vi "Get Named Range.vi"(7 "Sheet Name":string, 8 "error in":errorcluster, 10 "Range Identifier":string, 11 "SpreadsheetDoc in":refnum<k24>) -> (0 "error out":errorcluster, 2 "Range":string, 3 "SpreadsheetDoc out":refnum<k24>, 5 "Sheet Name":string)   [LabVIEW 2019, in "Open Xml.lvlib"]
uses:
  Open Xml.lvlib
  D:/git/Open-Xml-LabVIEW/Source/DocumentFormat.OpenXml.dll
  DocumentFormat.OpenXml.dll
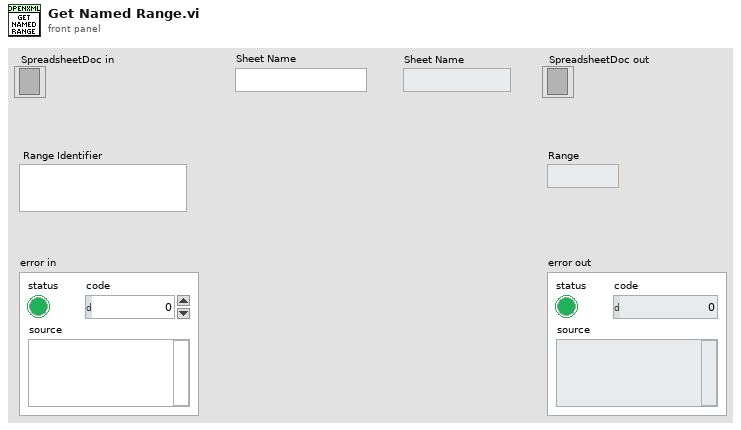
[diagram p1: front panel]
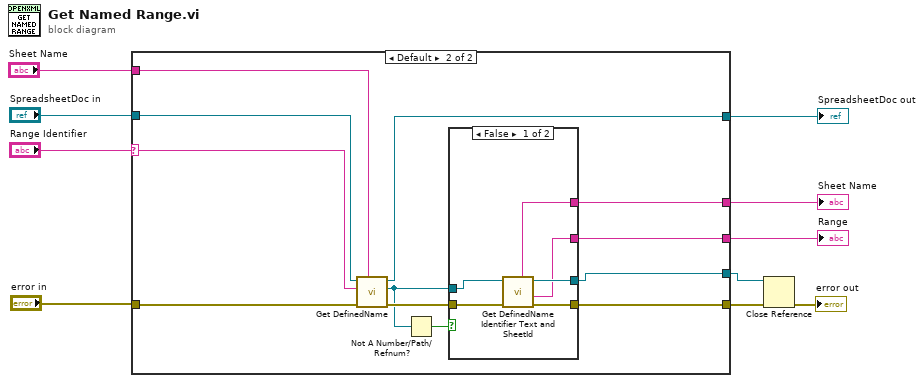
[diagram p0: block diagram]
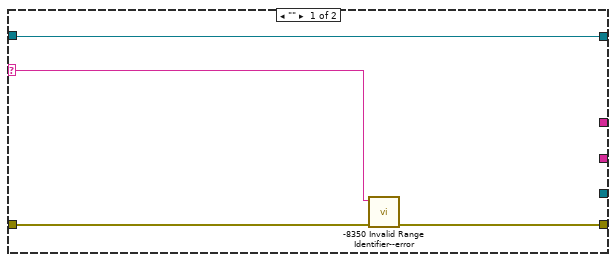
[diagram p2: hidden frame]
diagram:
  n1 = case shown="Default" "Range Identifier" {
    selector: "Range Identifier" -> [w12 w24]
    tunnel: "error in" -> [w14 w26]
    tunnel: [w13 w17] -> w10
    tunnel: "SpreadsheetDoc in" -> [w11 w20]
    tunnel: [w11 w19] -> w8
    tunnel: "Sheet Name" -> [_ w25]
    tunnel: [_ w18] -> w5
    tunnel: [_ w16] -> w4
    tunnel: [_ w15] -> w3
    frame "" {
      n2 = call "-8350 Invalid Range Identifier--error.vi"("error in"=w14, "Argument"=w12) -> ("error out"=w13:errorcluster)  [unwired: 9 in]
    }
    frame Default {
      n3 = call "Get DefinedName.vi"("Sheet Name"=w25, "error in"=w26, "Range Identifier"=w24, "SpreadsheetDoc in"=w20) -> ("error out"=w23:errorcluster, "DefinedName"=w21:refnum<k24>, "SpreadsheetDoc out"=w19:refnum<k24>)  [unwired: 4 in, 1 out]
      n4 = Not A Number/Path/Refnum?(number/path/refnum=w21) -> (NaN/Path/Refnum?=w22:bool)
      n5 = case shown="False" w22 {
        tunnel: [w32 w33] -> w15
        tunnel: w23 -> [w30 w34]
        tunnel: w21 -> [w31 w33]
        tunnel: [w29 w34] -> w17
        tunnel: [w28 _] -> w18
        tunnel: [w27 _] -> w16
        frame False {
          n6 = call "Get DefinedName Identifier Text and SheetId.vi"("error in"=w30, "DefinedName in"=w31) -> ("error out"=w29:errorcluster, "Range"=w27:string, "DefinedName out"=w32:refnum<k24>, "Sheet Name"=w28:string)  [unwired: 5 in, 1 out]
        }
        frame True {
        }
      }
    }
  }
  "SpreadsheetDoc out" <- w8
  "Sheet Name" <- w5
  "Range" <- w4
  n7 = Close Reference(reference=w3, error in (no error)=w10) -> (error out=→"error out":errorcluster)
